vi "getStatus_action.vi"(0 "HGF_ImaqFg":refnum<class "HGF_ImaqFg.lvclass">, 5 "error in (no error)":errorcluster) -> (13 "Lost Counter":T1, 14 "dup HGF_ImaqFg":refnum<class "HGF_ImaqFg.lvclass">, 15 "Acquiring?":bool, 16 "Last Valid Buffer Index":u32, 17 "Last Valid Buffer Number":u32, 19 "error out":errorcluster)   [LabVIEW 2014, in "HGF_IMAQ.lvlib" / "HGF_ImaqFg.lvclass"]
doc: "Returns status information about the acquisition, such as the state of the acquisition and the last valid buffer acquired."
uses:
  HGF_ImaqFg.lvclass
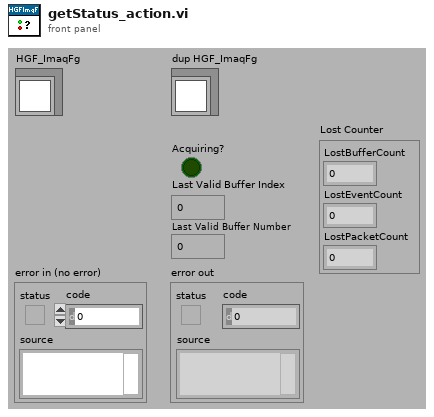
[diagram p1: front panel]
types:
  T1 = cluster{"LostBufferCount":u32, "LostEventCount":u32, "LostPacketCount":u32}
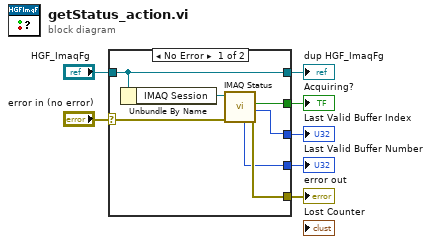
[diagram p0: block diagram]
diagram:
  n1 = case shown="No Error" "error in (no error)" {
    selector: "error in (no error)" -> [w9 w15]
    tunnel: [w14 w15] -> w7
    tunnel: [w13 _] -> w6
    tunnel: [w12 _] -> w5
    tunnel: [w11 _] -> w4
    tunnel: "HGF_ImaqFg" -> [w8 w16]
    tunnel: [w8 w16] -> w1
    frame No Error {
      n2 = Unbundle By Name(w8) -> ("IMAQ Session"=w10:refnum<k11>)
      n3 = call <vilib>:"IMAQ Status.vi"("error in (no error)"=w9, "IMAQ Session In"=w10) -> ("error out"=w14:errorcluster, "Last Valid Buffer Index"=w12:i32, "Acquiring?"=w13:bool, "Last Valid Buffer Number"=w11:i32)  [unwired: 5 in, 1 out]
    }
    frame Error {
    }
  }
  "error out" <- w7
  "dup HGF_ImaqFg" <- w1
  "Acquiring?" <- w6
  "Last Valid Buffer Index" <- w5
  "Last Valid Buffer Number" <- w4
